vi "Key Down Up Layers.vi"(8 "error in":errorcluster, 9 "Shift?":bool, 10 "VKey":T8, 11 "Data in":T1={"Class"={"Ants"=refnum, "Layer"=refnum, "Templates"=refnum, "Icon"=refnum, "Glyph"=refnum, "Settings"=refnum, "Tools"=refnum}, "Ref"={"Add Layer"=refnum, "Remove Layer"=refnum, "Line Text"=[], "Body Text Spec"=refnum, "DNL_Font"=refnum, "glyph path str"=refnum, "templates path str"=refnum, "Arrow Up"=refnum, "Arrow Down"=refnum, "IE VI Ref"=refnum, "Glyphs tree"=refnum, "Templates tree"=refnum, "Layer Icon Text"=refnum, "Layer Template"=refnum, "Clipboard"=refnum, "BW icon in"=refnum, "Color icon in"=refnum, "Layer Clust"=refnum, "Body Text"=refnum, "DNL_Framework Templates"=refnum, "Search Templates"=refnum, "TextMarker"=refnum, "Tab Control"=refnum, "Search Glyphs"=refnum, "Line Color"=refnum, "DNL_Glyphs []"=refnum, "Fill Color"=refnum, "Tools"=refnum, "Glyphs tree"=refnum, "Icon"=refnum, "Preview"=refnum, "Ants"=refnum, "Terminals"=refnum, "menu reference"=refnum, "LayerNames"=[], "GlyphLoadAnimation"=refnum, "TemplateLoadAnimation"=refnum, "refreshGlyphs"=refnum, "refreshTemplates"=refnum}, "Support"={"AntsRect"={"left"=0, "top"=0, "right"=0, "bottom"=0}, "Mouse Move Coords"={"Horizontal"=0, "Vertical"=0}, "Mouse Down Coords"={"Horizontal"=0, "Vertical"=0}, "Temp Coord"={"Horizontal"=0, "Vertical"=0}, "Action"=enum."Default", "Edge Color"=4914962, "Fill Color"=16860, "Mouse Down?"=FALSE, "Draft Mode?"=FALSE, "Temp Icon"=bytes[3102], "CTRL Pressed"=FALSE, "Move Selection?"=FALSE, "AntsRect Orig"={"left"=0, "top"=0, "right"=0, "bottom"=0}, "Text"="", "TM Set?"=FALSE, "Mouse inside icon?"=FALSE, "Tool (old value)"=0, "Pencil Move Color"=0, "Swap Colors?"=FALSE, "Shift pressed?"=FALSE}}) -> (0 "error out":errorcluster, 3 "Data out":T1={"Class"={"Ants"=refnum, "Layer"=refnum, "Templates"=refnum, "Icon"=refnum, "Glyph"=refnum, "Settings"=refnum, "Tools"=refnum}, "Ref"={"Add Layer"=refnum, "Remove Layer"=refnum, "Line Text"=[], "Body Text Spec"=refnum, "DNL_Font"=refnum, "glyph path str"=refnum, "templates path str"=refnum, "Arrow Up"=refnum, "Arrow Down"=refnum, "IE VI Ref"=refnum, "Glyphs tree"=refnum, "Templates tree"=refnum, "Layer Icon Text"=refnum, "Layer Template"=refnum, "Clipboard"=refnum, "BW icon in"=refnum, "Color icon in"=refnum, "Layer Clust"=refnum, "Body Text"=refnum, "DNL_Framework Templates"=refnum, "Search Templates"=refnum, "TextMarker"=refnum, "Tab Control"=refnum, "Search Glyphs"=refnum, "Line Color"=refnum, "DNL_Glyphs []"=refnum, "Fill Color"=refnum, "Tools"=refnum, "Glyphs tree"=refnum, "Icon"=refnum, "Preview"=refnum, "Ants"=refnum, "Terminals"=refnum, "menu reference"=refnum, "LayerNames"=[], "GlyphLoadAnimation"=refnum, "TemplateLoadAnimation"=refnum, "refreshGlyphs"=refnum, "refreshTemplates"=refnum}, "Support"={"AntsRect"={"left"=0, "top"=0, "right"=0, "bottom"=0}, "Mouse Move Coords"={"Horizontal"=0, "Vertical"=0}, "Mouse Down Coords"={"Horizontal"=0, "Vertical"=0}, "Temp Coord"={"Horizontal"=0, "Vertical"=0}, "Action"=enum."Default", "Edge Color"=4914962, "Fill Color"=16860, "Mouse Down?"=FALSE, "Draft Mode?"=FALSE, "Temp Icon"=bytes[3102], "CTRL Pressed"=FALSE, "Move Selection?"=FALSE, "AntsRect Orig"={"left"=0, "top"=0, "right"=0, "bottom"=0}, "Text"="", "TM Set?"=FALSE, "Mouse inside icon?"=FALSE, "Tool (old value)"=0, "Pencil Move Color"=0, "Swap Colors?"=FALSE, "Shift pressed?"=FALSE}})   [LabVIEW 2021]
uses:
  <vilib>/event_ctls.llb/eventvkey.ctl
  <resource>/plugins/NIIconEditor/Controls/IE Data.ctl
  <resource>/plugins/NIIconEditor/Class/Ants/Ants.lvclass
  <resource>/plugins/NIIconEditor/Class/FakedArray/FakedArray.lvclass
  <resource>/plugins/NIIconEditor/Class/Icon Library/Glyph.lvclass
  <resource>/plugins/NIIconEditor/Class/Settings/Settings.lvclass
  <resource>/plugins/NIIconEditor/Class/Tools/Tools Paint.lvclass
  <vilib>/LabVIEW Icon API/lv_icon/Classes/Icon/Icon.lvclass
  <resource>/plugins/NIIconEditor/Controls/IE Classes.ctl
  <resource>/plugins/NIIconEditor/Controls/References Cluster.ctl
  <resource>/plugins/NIIconEditor/Controls/SupportClass.ctl
  <vilib>/Utility/miscctls.llb/LVPoint32TypeDef.ctl
  <resource>/plugins/NIIconEditor/Controls/SupportClass_Action.ctl
  <vilib>/LabVIEW Icon API/lv_icon/Controls/IEColor.ctl
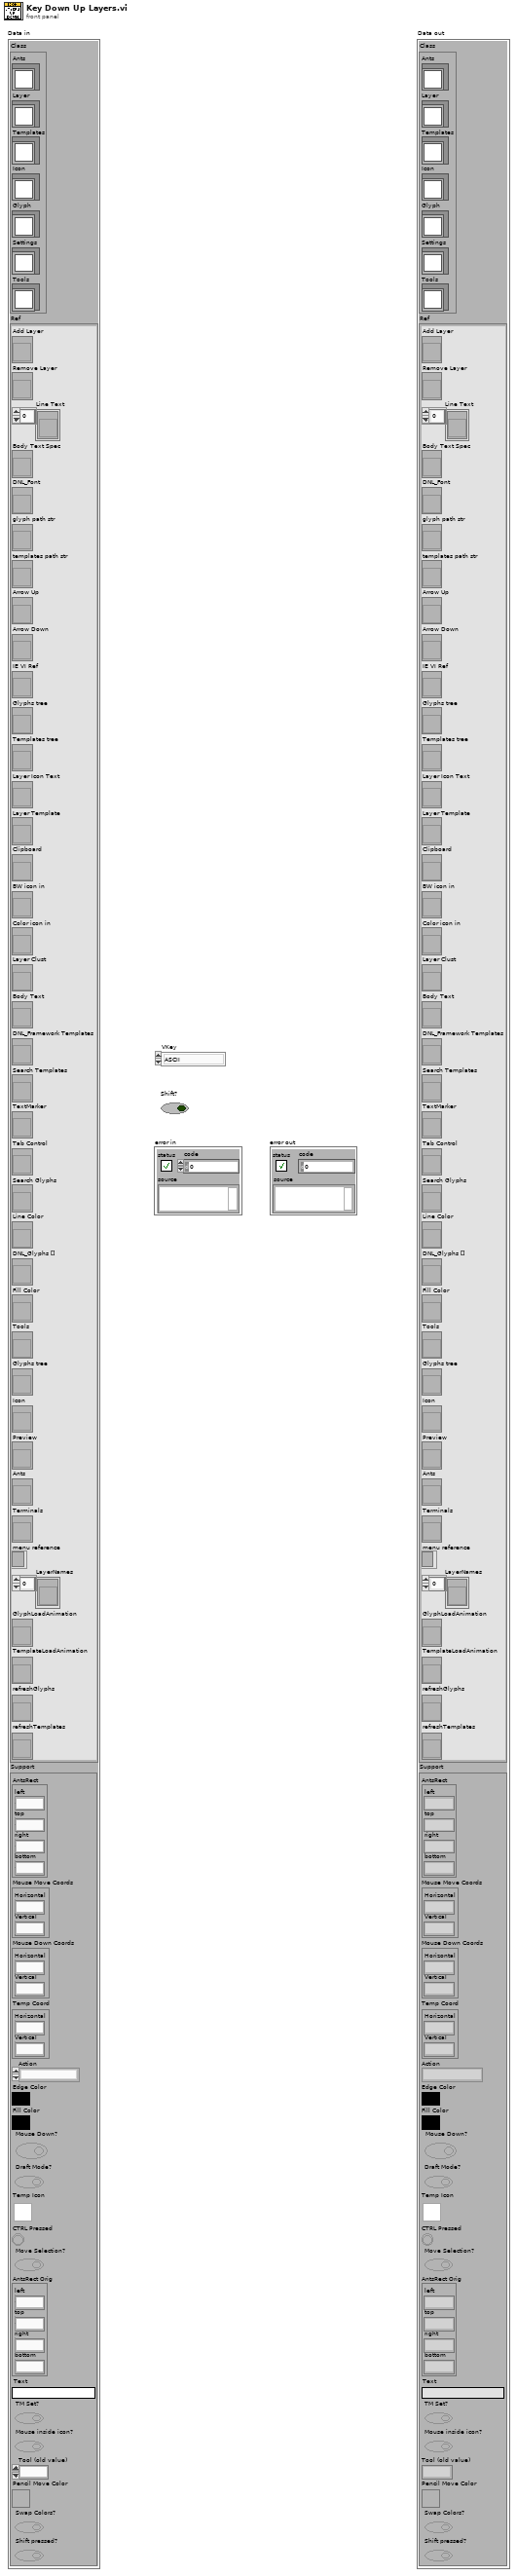
[diagram p1: front panel]
types:
  T1 = typedef "IE Data.ctl" = cluster{"Class":T2, "Ref":T3, "Support":T4}
  T2 = typedef "IE Classes.ctl" = cluster{"Ants":refnum<class "Ants.lvclass">, "Layer":refnum<class "FakedArray.lvclass">, "Templates":refnum<class "FakedArray.lvclass">, "Icon":refnum<class "Icon.lvclass">, "Glyph":refnum<class "Glyph.lvclass">, "Settings":refnum<class "Settings.lvclass">, "Tools":refnum<class "Tools Paint.lvclass">}
  T3 = typedef "References Cluster.ctl" = cluster{"Add Layer":refnum<vi>, "Remove Layer":refnum<vi>, "Line Text":refnum<vi>[], "Body Text Spec":refnum<vi>, "DNL_Font":refnum<vi>, "glyph path str":refnum<vi>, "templates path str":refnum<vi>, "Arrow Up":refnum<vi>, "Arrow Down":refnum<vi>, "IE VI Ref":refnum<vi>, "Glyphs tree":refnum<vi>, "Templates tree":refnum<vi>, "Layer Icon Text":refnum<vi>, "Layer Template":refnum<vi>, "Clipboard":refnum<vi>, "BW icon in":refnum<vi>, "Color icon in":refnum<vi>, "Layer Clust":refnum<vi>, "Body Text":refnum<vi>, "DNL_Framework Templates":refnum<vi>, "Search Templates":refnum<vi>, "TextMarker":refnum<vi>, "Tab Control":refnum<vi>, "Search Glyphs":refnum<vi>, "Line Color":refnum<vi>, "DNL_Glyphs []":refnum<vi>, "Fill Color":refnum<vi>, "Tools":refnum<vi>, "Glyphs tree":refnum<vi>, "Icon":refnum<vi>, "Preview":refnum<vi>, "Ants":refnum<vi>, "Terminals":refnum<vi>, "menu reference":refnum<k9>, "LayerNames":refnum<vi>[], "GlyphLoadAnimation":refnum<vi>, "TemplateLoadAnimation":refnum<vi>, "refreshGlyphs":refnum<vi>, "refreshTemplates":refnum<vi>}
  T4 = typedef "SupportClass.ctl" = cluster{"AntsRect":cluster{"left":i16, "top":i16, "right":i16, "bottom":i16}, "Mouse Move Coords":T5, "Mouse Down Coords":T5, "Temp Coord":T5, "Action":T6, "Edge Color":T7, "Fill Color":T7, "Mouse Down?":bool, "Draft Mode?":bool, "Temp Icon":picture, "CTRL Pressed":bool, "Move Selection?":bool, "AntsRect Orig":cluster{"left":i16, "top":i16, "right":i16, "bottom":i16}, "Text":string, "TM Set?":bool, "Mouse inside icon?":bool, "Tool (old value)":u32, "Pencil Move Color":u32, "Swap Colors?":bool, "Shift pressed?":bool}
  T5 = typedef "LVPoint32TypeDef.ctl" = cluster{"Horizontal":i32, "Vertical":i32}
  T6 = typedef "SupportClass_Action.ctl" = enum16{"Default", "Move Selection", "Glyph Library", "Tool"}
  T7 = typedef "IEColor.ctl" = u32
  T8 = typedef "eventvkey.ctl" = enum16{"ASCII", "Enter", "Return", "Shift", "Ctrl", "Alt", "Cmd", "Opt", "Caps", "NumLock", "Clear", "Break", "Up", "Down", "Left", "Right", "Insert", "Delete", "Home", "End", "PageUp", "PageDown", "Escape", "Help", "Pause", "ScrollLock", "F1", "F2", "F3", "F4", "F5", "F6", "F7", "F8", "F9", "F10", "F11", "F12", "F13", "F14", "F15", "F16", "F17", "F18", "F19", "F20", "F21", "F22", "F23", "F24", "Play", "VolumeUp", "VolumeDown", "Mute", "Two Byte Char"}
  T9 = enum32{"Templates", "Icon Text", "Glyphs", "Layers"}
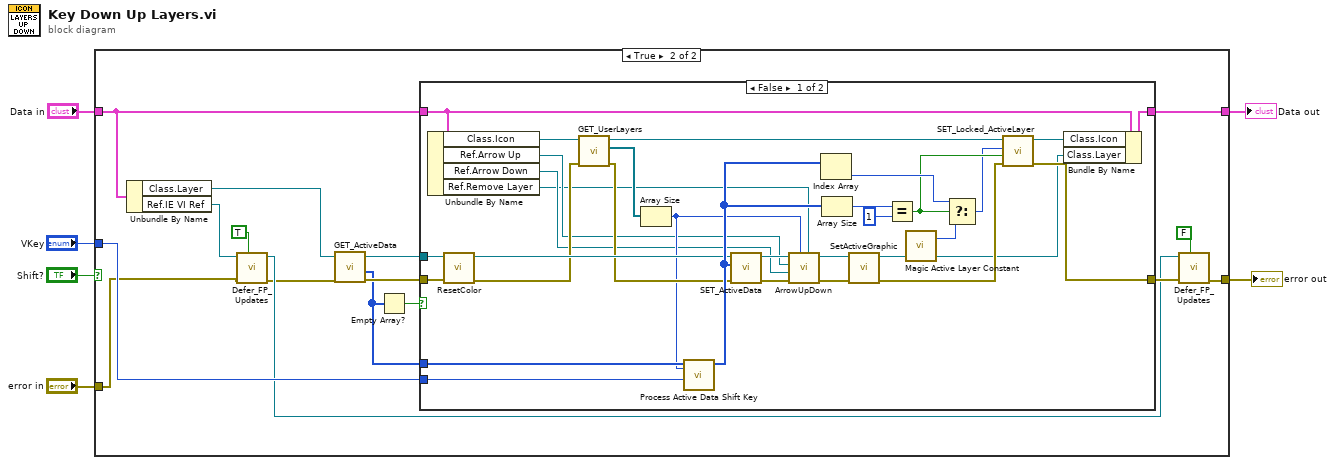
[diagram p0: block diagram]
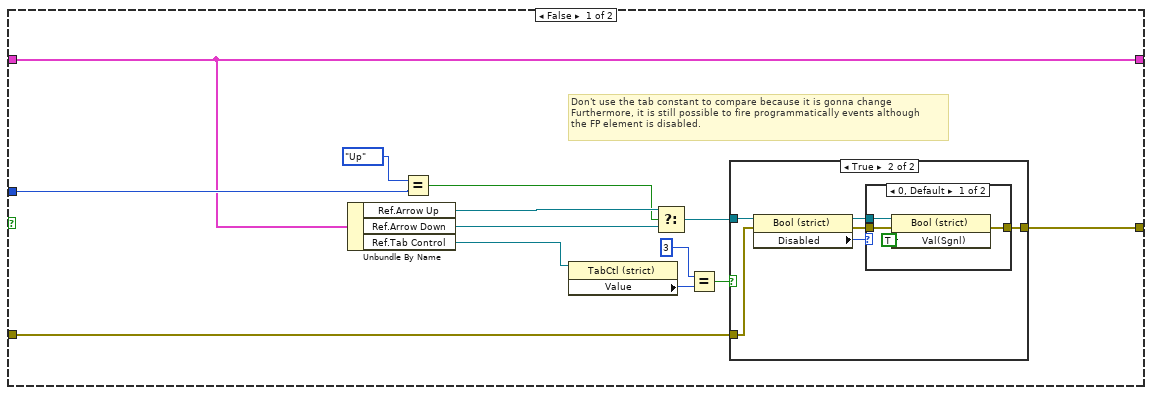
[diagram p2: hidden frame]
diagram:
  n1 = case shown="True" "Shift?" {
    tunnel: [w19 w41] -> w6
    tunnel: "error in" -> [w18 w37]
    tunnel: "VKey" -> [w9 w42]
    tunnel: "Data in" -> [w7 w33]
    tunnel: [w7 w32] -> w1
    frame False {
      # "Don't use the tab constant to compare because it is gonna change\nFurthermore, it is still possible to fire programmatically events although\nthe FP element is disabled."
      n2 = Unbundle By Name(w7) -> ("Ref.Arrow Up"=w14:refnum<vi>, "Ref.Arrow Down"=w13:refnum<vi>, "Ref.Tab Control"=w15:refnum<vi>)
      n3 = Equal?(x=eventvkey."Up", y=w9) -> (x = y?=w8:bool)
      n4 = property class="TabCtl (strict)"(reference=w15) -> ("Value"=w16:T9)  [unwired: 1 in, 2 out]
      n5 = Select(t=w14, s=w8, f=w13) -> (s? t:f=w12:refnum<vi>)
      n6 = Equal?(x=u32 3, y=w16) -> (x = y?=w11:bool)
      n7 = case shown="True" w11 {
        tunnel: w18 -> [w20 w22]
        tunnel: [w20 w26] -> w19
        tunnel: w12 -> [_ w23]
        frame False {
        }
        frame True {
          n8 = property class="Bool (strict)"(reference=w23, error in=w22) -> (reference out=w24:refnum<vi>, error out=w21:errorcluster, "Disabled"=w25:u8)
          n9 = case shown="0, Default" w25 {
            tunnel: [w29 w31] -> w26
            tunnel: w24 -> [w28 _]
            tunnel: w21 -> [w27 w31]
            frame 0, Default {
              n10 = property class="Bool (strict)"(reference=w28, error in=w27, "Val(Sgnl)"=TRUE) -> (error out=w29:errorcluster)  [unwired: 1 out]
            }
            frame 2 {
            }
          }
        }
      }
    }
    frame True {
      n11 = Unbundle By Name(w33) -> ("Class.Layer"=w35:refnum<class "FakedArray.lvclass">, "Ref.IE VI Ref"=w36:refnum<vi>)
      n12 = call <resource>:"Defer_FP_Updates.vi"("Defer Panel Updates"=TRUE, "error in (no error)"=w37, "lv_icon.vi in"=w36) -> ("error out"=w34:errorcluster, "lv icon.vi out"=w39:refnum<vi>)  [unwired: 7 out]
      n13 = call-dynamic "GET_ActiveData.vi"("error in (no error)"=w34, "FakedArray in"=w35) -> ("error out"=w45:errorcluster, "Active Data []"=w43:i32[], "FakedArray out"=w44:refnum<class "FakedArray.lvclass">)  [unwired: 7 out]
      n14 = Empty Array?(array=w43) -> (empty?=w46:bool)
      n15 = case shown="False" w46 {
        tunnel: [w54 w80] -> w40
        tunnel: w45 -> [w72 w80]
        tunnel: w44 -> [w71 _]
        tunnel: w43 -> [w67 _]
        tunnel: w42 -> [w68 _]
        tunnel: w33 -> [w55 w79]
        tunnel: [w52 w79] -> w32
        frame False {
          n16 = Unbundle By Name(w55) -> ("Class.Icon"=w58:refnum<class "Icon.lvclass">, "Ref.Arrow Up"=w49:refnum<vi>, "Ref.Arrow Down"=w50:refnum<vi>, "Ref.Remove Layer"=w48:refnum<vi>)
          n17 = call <resource>:"ResetColor.vi"("error in (no error)"=w72, "FakedArray in"=w71) -> ("error out"=w57:errorcluster, "FakedArray out"=w61:refnum<class "FakedArray.lvclass">)  [unwired: 8 out]
          n18 = call-dynamic "GET_UserLayers.vi"("error in (no error)"=w57, "Icon.lvclass in"=w58) -> ("error out"=w60:errorcluster, "All Layers"=w70:refnum<class "Layer.lvclass">[], "Icon.lvclass out"=w69:refnum<class "Icon.lvclass">)  [unwired: 7 out]
          n19 = Array Size(array=w70) -> (size(s)=w59:i32)
          n20 = call <resource>:"Process Active Data Shift Key.vi"("# User Layers"=w59, "VKey"=w68, "Active Data [] in"=w67) -> ("Active Data [] out"=w66:i32[])  [unwired: 8 out]
          n21 = call-dynamic "SET_ActiveData.vi"("error in (no error)"=w60, "Active Data"=w66, "FakedArray.lvclass in"=w61) -> ("error out"=w65:errorcluster, "FakedArray.lvclass out"=w62:refnum<class "FakedArray.lvclass">)  [unwired: 7 out]
          n22 = call <resource>:"ArrowUpDown.vi"("Remove Layer"=w48, "# Layers"=w59, "error in (no error)"=w65, "Arrow Down"=w50, "Arrow Up"=w49, "FakedArray in"=w62) -> ("error out"=w64:errorcluster, "FakedArray out"=w63:refnum<class "FakedArray.lvclass">)  [unwired: 4 out]
          n23 = Index Array(array=w66) -> (element=w76:i32)  [unwired: 1 in]
          n24 = Array Size(array=w66) -> (size(s)=w78:i32)
          n25 = call-dynamic "SetActiveGraphic.vi"("error in (no error)"=w64, "FakedArray in"=w63) -> ("error out"=w53:errorcluster, "FakedArray out"=w51:refnum<class "FakedArray.lvclass">)  [unwired: 4 in, 4 out]
          n26 = Equal?(x=w78, y=1) -> (x = y?=w75:bool)
          n27 = call <resource>:"Magic Active Layer Constant.vi"() -> ("Magic Constant"=w74:i32)  [unwired: 19 out]
          n28 = Select(t=w76, s=w75, f=w74) -> (s? t:f=w73:i32)
          n29 = call-dynamic "SET_Locked_ActiveLayer.vi"("error in (no error)"=w53, "Layers Locked?"=w75, "Active Layer"=w73, "Icon.lvclass in"=w69) -> ("error out"=w54:errorcluster, "Icon.lvclass out"=w56:refnum<class "Icon.lvclass">)  [unwired: 6 in]
          n30 = Bundle By Name(cluster=w55, "Class.Icon"=w56, "Class.Layer"=w51) -> (w52:T1)
        }
        frame True {
        }
      }
      n31 = call <resource>:"Defer_FP_Updates.vi"("Defer Panel Updates"=FALSE, "error in (no error)"=w40, "lv_icon.vi in"=w39) -> ("error out"=w41:errorcluster)  [unwired: 8 out]
    }
  }
  "error out" <- w6
  "Data out" <- w1
